vi "BypassControl.vi"(6 "Cutoff":dbl=0.15 format="%#_13g", 8 "AccelRate":dbl, 9 "LoopTime":dbl, 10 "DesiredInput":dbl, 11 "CurrentInput":dbl) -> (3 "SetMotor":dbl)   [LabVIEW 2013]
doc: "Skips motor values that are, for all intents and purposes, 0. This VI includes trapezoidal acceleration."
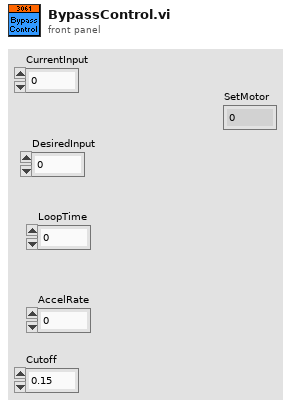
[diagram p1: front panel]
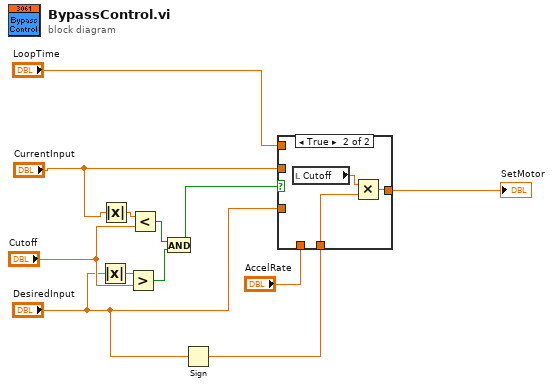
[diagram p0: block diagram]
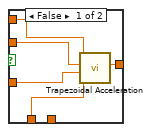
[diagram p2: hidden frame]
diagram:
  n1 = Absolute Value(x="DesiredInput") -> (abs(x)=w10:dbl)
  n2 = Absolute Value(x="CurrentInput") -> (abs(x)=w11:dbl)
  n3 = Greater?(x=w10, y="Cutoff") -> (0:w8:bool)
  n4 = Less?(x=w11, y="Cutoff") -> (x < y?=w9:bool)
  n5 = And(x=w9, y=w8) -> (x .and. y?=w7:bool)
  n6 = Sign(1:"DesiredInput") -> (0:w5:dbl)
  n7 = case shown="True" w7 {
    tunnel: "DesiredInput" -> [w16 _]
    tunnel: "CurrentInput" -> [w17 _]
    tunnel: [w15 w20] -> w4
    tunnel: w5 -> [_ w19]
    tunnel: "LoopTime" -> [w14 _]
    tunnel: "AccelRate" -> [w13 _]
    frame False {
      n8 = call "Trapezoidal Acceleration.vi"("AccelRate"=w13, "Desired"=w16, "Actual"=w17, "LoopTime"=w14) -> ("New Actual"=w15:dbl)  [unwired: 7 in]
    }
    frame True {
      n9 = local read "Cutoff"() -> (w18:dbl)
      n10 = Multiply(x=w18, y=w19) -> (x*y=w20:dbl)
    }
  }
  "SetMotor" <- w4
